vi "Read Configuration Parameters.vi"(8 "error in (no error)":errorcluster, 10 "refnum":T1, 11 "HW with output config in":refnum<class "HW with output config.lvclass">) -> (0 "error out":errorcluster, 2 "refnum out":T1, 3 "HW with output config out":refnum<class "HW with output config.lvclass">)   [LabVIEW 2026, in "Hardware.lvlib" / "HW with output config.lvclass"]
uses:
  HW with output config.lvclass
  <vilib>/Utility/config.llb/Config Data RefNum.ctl
  configuration/Configuration.lvclass/Configuration.ctl
  HW with output config.lvclass/HW with output config.ctl
  HW Config/HW Configuration.lvclass
  configuration/Configuration.lvclass
  <vilib>/Utility/config.llb/NI_LVConfig.lvlib
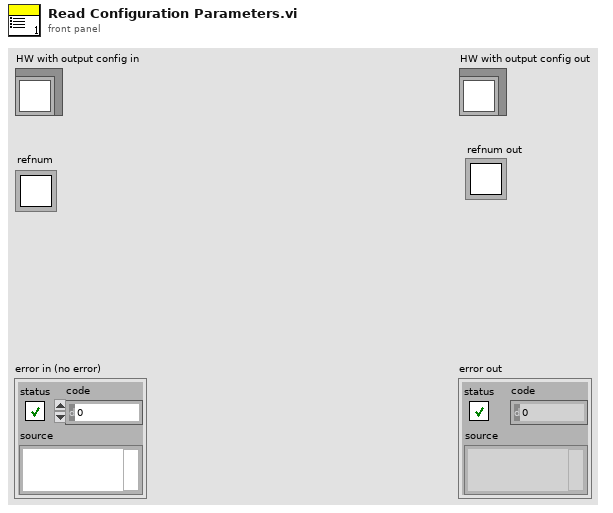
[diagram p1: front panel]
types:
  T1 = typedef "NI_LVConfig.lvlib/Config Data RefNum.ctl" = refnum<k1>
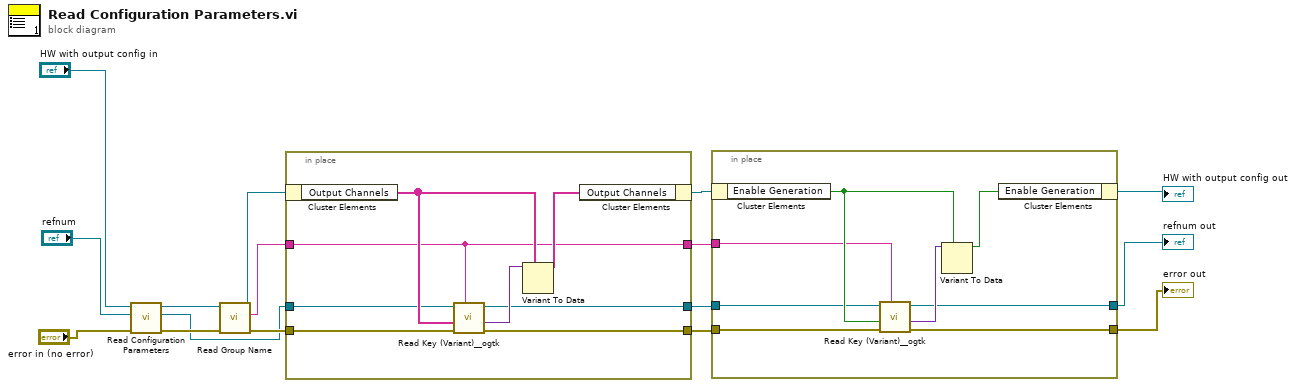
[diagram p0: block diagram]
diagram:
  n1 = call-parent "Read Configuration Parameters.vi"("error in (no error)"="error in (no error)", "refnum"="refnum", "HW Configuration in"="HW with output config in") -> ("error out"=w3:errorcluster, "refnum out"=w1:T1, "HW Configuration out"=w12:refnum<class "HW with output config.lvclass">)  [unwired: 6 in]
  n2 = call "Read Group Name.vi"("error in (no error)"=w3, "Configuration in"=w12) -> ("error out"=w4:errorcluster, "Group Name"=w14:string, "Configuration out"=w13:refnum<class "HW with output config.lvclass">)  [unwired: 7 in]
  n3 = in-place {
    in-place-border: w1 -> [w21]
    in-place-border: [w20] -> w9
    in-place-border: w4 -> [w19]
    in-place-border: [w18] -> w8
    in-place-border: w14 -> [w17]
    in-place-border: [w17] -> w10
    n4 = in-place-cluster #1(w13) -> ("Output Channels"=w24:string[])
    n5 = call <userlib>:"Read Key (Variant)__ogtk.vi"("section"=w17, "error in (no error)"=w19, "type"=w24, "refnum"=w21) -> ("error out"=w18:errorcluster, "key-value"=w23:variant, "refnum out"=w20:T1)  [unwired: 4 in, 1 out]
    n6 = Variant To Data(type=w24, Variant=w23) -> (data=w22:string[])  [unwired: 1 in, 1 out]
    n7 = in-place-cluster #1("Output Channels"=w22) -> (w11:refnum<class "HW with output config.lvclass">)
  }
  n8 = in-place {
    in-place-border: w9 -> [w29]
    in-place-border: [w28] -> w7
    in-place-border: w8 -> [w27]
    in-place-border: [w26] -> w5
    in-place-border: w10 -> [w25]
    n9 = in-place-cluster #2(w11) -> ("Enable Generation"=w32:bool)
    n10 = call <userlib>:"Read Key (Variant)__ogtk.vi"("section"=w25, "error in (no error)"=w27, "type"=w32, "refnum"=w29) -> ("error out"=w26:errorcluster, "key-value"=w31:variant, "refnum out"=w28:T1)  [unwired: 4 in, 1 out]
    n11 = Variant To Data(type=w32, Variant=w31) -> (data=w30:bool)  [unwired: 1 in, 1 out]
    n12 = in-place-cluster #2("Enable Generation"=w30) -> (→"HW with output config out":refnum<class "HW with output config.lvclass">)
  }
  "error out" <- w5
  "refnum out" <- w7
